vi "_emi_Loop index generator.vi"(11 "error in (no error)":errorcluster) -> (8 "Loop ID out":u16, 15 "error out":errorcluster)   [LabVIEW 2010]
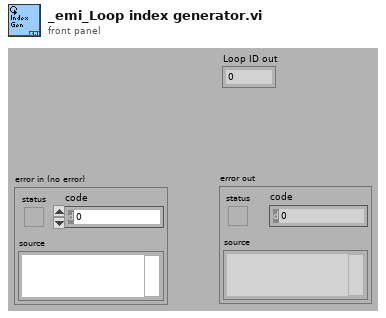
[diagram p1: front panel]
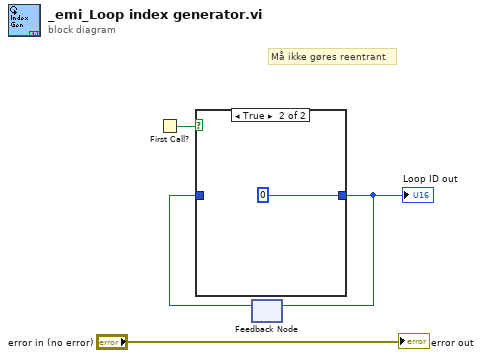
[diagram p0: block diagram]
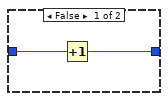
[diagram p2: hidden frame]
diagram:
  # "Må ikke gøres reentrant"
  n1 = First Call?() -> (First Call?: T/F=w2:bool)
  n2 = feedback #1() -> (w3:u16)  [unwired: 1 in]
  n3 = case shown="True" w2 {
    tunnel: w3 -> [w6 _]
    tunnel: [w5 u16 0 ("Loop ID")] -> w1
    frame False {
      n4 = Increment(x=w6) -> (x+1=w5:u16)
    }
    frame True {
    }
  }
  "Loop ID out" <- w1
  n5 = feedback-in #1(w1) -> ()
  "error out" <- "error in (no error)"
